vi "atomNumberWolf.vi"(6 "Image bg":sgl[][](array[numeric]) format="%.2f", 8 "error in (no error)":errorcluster, 9 "Image ref":sgl[][](array[numeric]) format="%.2f", 10 "Image object":sgl[][](array[numeric]) format="%.2f", 11 "BECImageProcessor in":refnum<class "BECImageProcessor.lvclass">) -> (0 "error out":errorcluster, 1 "z width":dbl, 2 "number":dbl, 3 "BECImageProcessor out":refnum<class "BECImageProcessor.lvclass">)   [LabVIEW 2009, in "Tools.lvlib" / "Imaging.lvlib" / "BECImageProcessor.lvclass"]
uses:
  BECImageProcessor.lvclass
  <vilib>/Analysis/NI_AALBase.lvlib
panel:
  out "x width":dbl
  out "XY Graph":cluster{i32[], dbl[]}(graph)
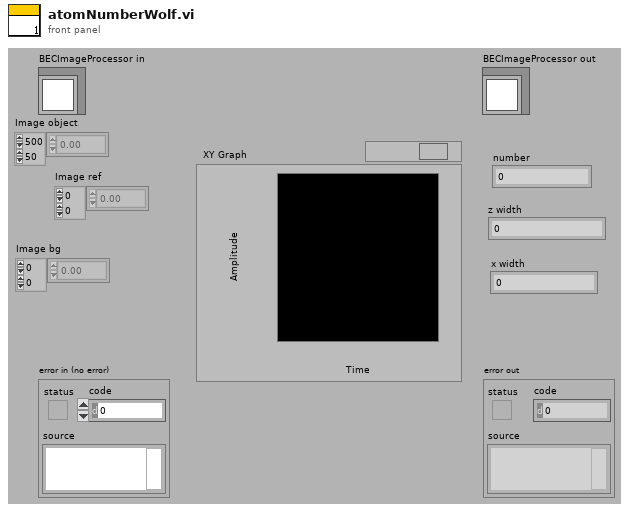
[diagram p1: front panel]
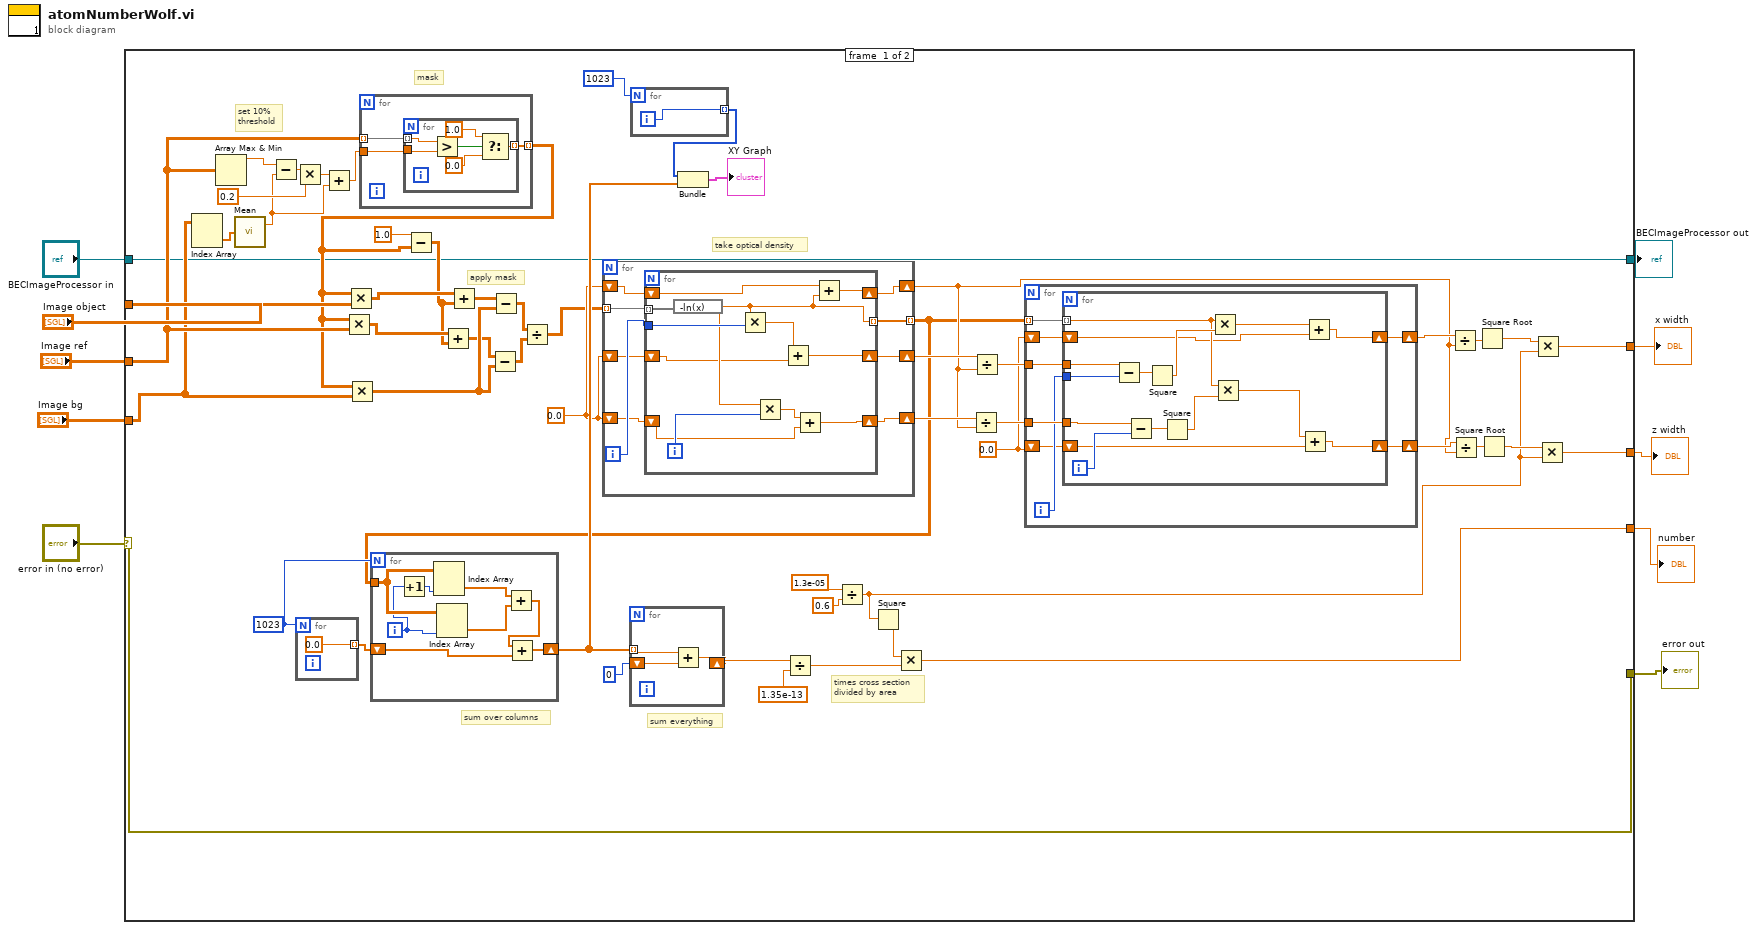
[diagram p0: block diagram]
diagram:
  n1 = case shown="No Error" "error in (no error)" {
    selector: "error in (no error)" -> [w64 w132]
    tunnel: [w64 w132] -> w9
    tunnel: [w15 w131] -> w7
    tunnel: "BECImageProcessor in" -> [w15 w131]
    tunnel: "Image object" -> [w53 _]
    tunnel: "Image ref" -> [w51 _]
    tunnel: "Image bg" -> [w39 _]
    tunnel: [w56 _] -> w3
    tunnel: [w17 _] -> w2
    tunnel: [w16 _] -> w1
    frame #0 {
      w26 = 0.0
      w31 = 0.0
      w55 = 1023
      # "set 10%\nthreshold"
      # "apply mask"
      # "mask"
      # "times cross section\ndivided by area"
      # "sum everything"
      # "sum over columns"
      # "take optical density"
      n2 = Index Array(array=w39) -> (element=w38:sgl[])  [unwired: 2 in]
      n3 = Array Max & Min(array=w51) -> (max value=w37:sgl)  [unwired: 3 out]
      n4 = call <vilib>:"Mean.vi"("X"=w38) -> ("mean"=w33:dbl)  [unwired: 1 out]
      n5 = Subtract(x=w37, y=w33) -> (x-y=w36:dbl)
      n6 = Multiply(x=w36, y=0.2) -> (x*y=w34:dbl)
      n7 = for {
        N: w55 -> [_]
        tunnel: [0.0] -> w63 mode=indexing
      }
      n8 = Add(x=w34, y=w33) -> (x+y=w32:dbl)
      n9 = for {
        tunnel: w51 -> [w91] mode=indexing
        tunnel: [w90] -> w43 mode=indexing
        tunnel: w32 -> [w89]
        n10 = for {
          tunnel: w91 -> [w97] mode=indexing
          tunnel: w89 -> [w96]
          tunnel: [w92] -> w90 mode=indexing
          n11 = Greater?(x=w97, y=w96) -> (0:w95:bool)
          n12 = Select(t=1.0, s=w95, f=0.0) -> (s? t:f=w92:dbl)
        }
      }
      n13 = Multiply(x=w43, y=w51) -> (x*y=w42:dbl[][])
      n14 = Multiply(x=w43, y=w53) -> (x*y=w45:dbl[][])
      n15 = Multiply(x=w43, y=w39) -> (x*y=w52:dbl[][])
      n16 = Subtract(x=1.0, y=w43) -> (x-y=w41:dbl[][])
      n17 = Add(x=w42, y=w41) -> (x+y=w40:dbl[][])
      n18 = Add(x=w45, y=w41) -> (x+y=w46:dbl[][])
      n19 = Subtract(x=w40, y=w52) -> (x-y=w12:dbl[][])
      n20 = Subtract(x=w46, y=w52) -> (x-y=w11:dbl[][])
      n21 = Divide(x=w11, y=w12) -> (x/y=w13:dbl[][])
      n22 = for {
        tunnel: w13 -> [w109] mode=indexing
        tunnel: [w108] -> w14 mode=indexing
        shift-right: [w105] -> w29
        shift-left: w31 -> [w106]
        shift-right: [w103] -> w23
        shift-left: w31 -> [w104]
        shift-right: [w101] -> w30
        shift-left: w31 -> [w102]
        i -> [w107]
        n23 = for {
          tunnel: w109 -> [w121] mode=indexing
          tunnel: [w113] -> w108 mode=indexing
          tunnel: w107 -> [w120]
          shift-right: [w116] -> w105
          shift-left: w106 -> [w117]
          shift-right: [w115] -> w103
          shift-left: w104 -> [w114]
          shift-right: [w111] -> w101
          shift-left: w102 -> [w110]
          i -> [w119]
          n24 = expression code="-ln(x)"(w121) -> (w113:dbl)
          n25 = Multiply(x=w113, y=w120) -> (x*y=w112:dbl)
          n26 = Multiply(x=w113, y=w119) -> (x*y=w118:dbl)
          n27 = Add(x=w112, y=w110) -> (x+y=w111:dbl)
          n28 = Add(x=w118, y=w117) -> (x+y=w116:dbl)
          n29 = Add(x=w114, y=w113) -> (x+y=w115:dbl)
        }
      }
      n30 = for {
        N: w55 -> [_]
        tunnel: w14 -> [w130]
        shift-right: [w125] -> w47
        shift-left: w63 -> [w126]
        i -> [w123]
        n31 = Increment(x=w123) -> (x+1=w124:i32)
        n32 = Index Array(array=w130, index (col)=w124) -> (element=w129:dbl[])  [unwired: 1 in]
        n33 = Index Array(array=w130, index (col)=w123) -> (element=w128:dbl[])  [unwired: 1 in]
        n34 = Add(x=w129, y=w128) -> (x+y=w127:dbl[])
        n35 = Add(x=w127, y=w126) -> (x+y=w125:dbl[])
      }
      n36 = for {
        tunnel: w47 -> [w100] mode=indexing
        shift-right: [w99] -> w59
        shift-left: 0 -> [w98]
        n37 = Add(x=w100, y=w98) -> (x+y=w99:dbl)
      }
      n38 = for {
        N: 1023 -> [_]
        tunnel: [w88] -> w48 mode=indexing
        i -> [w88]
      }
      n39 = Bundle(w48, w47) -> (→"XY Graph":cluster{i32[], dbl[]})  [unwired: 1 in]
      n40 = Divide(x=w59, y=1.35e-13) -> (x/y=w57:dbl)
      n41 = Divide(x=1.3e-05, y=0.6) -> (x/y=w18:dbl)
      n42 = Square(x=w18) -> (x^2=w54:dbl)
      n43 = Multiply(x=w54, y=w57) -> (x*y=w56:dbl)
      n44 = Divide(x=w29, y=w23) -> (x/y=w28:dbl)
      n45 = Divide(x=w30, y=w23) -> (x/y=w27:dbl)
      n46 = for {
        tunnel: w28 -> [w72]
        tunnel: w27 -> [w71]
        tunnel: w14 -> [w70] mode=indexing
        shift-right: [w67] -> w24
        shift-left: w26 -> [w68]
        shift-right: [w65] -> w25
        shift-left: w26 -> [w66]
        i -> [w69]
        n47 = for {
          tunnel: w72 -> [w86]
          tunnel: w71 -> [w87]
          tunnel: w70 -> [w81] mode=indexing
          tunnel: w69 -> [w85]
          shift-right: [w76] -> w67
          shift-left: w68 -> [w77]
          shift-right: [w73] -> w65
          shift-left: w66 -> [w74]
          i -> [w84]
          n48 = Subtract(x=w87, y=w85) -> (x-y=w83:dbl)
          n49 = Subtract(x=w86, y=w84) -> (x-y=w80:dbl)
          n50 = Square(x=w83) -> (x^2=w82:dbl)
          n51 = Square(x=w80) -> (x^2=w79:dbl)
          n52 = Multiply(x=w81, y=w82) -> (x*y=w75:dbl)
          n53 = Multiply(x=w81, y=w79) -> (x*y=w78:dbl)
          n54 = Add(x=w78, y=w77) -> (x+y=w76:dbl)
          n55 = Add(x=w75, y=w74) -> (x+y=w73:dbl)
        }
      }
      n56 = Divide(x=w25, y=w23) -> (x/y=w22:dbl)
      n57 = Divide(x=w24, y=w23) -> (x/y=w21:dbl)
      n58 = Square Root(x=w22) -> (sqrt(x)=w20:dbl)
      n59 = Square Root(x=w21) -> (sqrt(x)=w19:dbl)
      n60 = Multiply(x=w20, y=w18) -> (x*y=w16:dbl)
      n61 = Multiply(x=w19, y=w18) -> (x*y=w17:dbl)
    }
    frame #1 {
    }
  }
  "error out" <- w9
  "BECImageProcessor out" <- w7
  "z width" <- w2
  "number" <- w3
  "x width" <- w1
